vi "PUT Actuation Direction.vi"(0 "Actuation Mode":T1) -> ()   [LabVIEW 2013]
uses:
  Action.ctl
  Experimental Parameters FGV Selector.ctl
  Actuation Mode.ctl
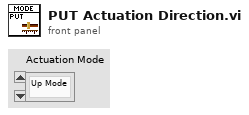
[diagram p1: front panel]
types:
  T1 = typedef "Actuation Mode.ctl" = enum16{"Up Mode", "Down Mode"}
  T2 = typedef "Experimental Parameters FGV Selector.ctl" = enum16{"Number of Samples", "Actuation Direction", "Ramp Rate", "Z Scan Size"}
  T3 = typedef "Action.ctl" = enum16{"GET", "PUT", "DELETE"}
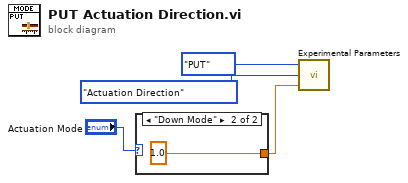
[diagram p0: block diagram]
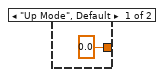
[diagram p2: hidden frame]
diagram:
  n1 = case shown="\"Down Mode\"" "Actuation Mode" {
    tunnel: [0.0 1.0] -> w1
    frame "Up Mode", Default {
    }
    frame "Down Mode" {
    }
  }
  n2 = call "Experimental Parameters.vi"("Input"=w1, "Experimental Parameters FGV Selector"=Experimental_Parameters_FGV_Selector."Actuation Direction", "Action"=Action."PUT") -> ()  [unwired: 1 out]
